vi "Perform Action.vi"(8 "error in":errorcluster, 10 "Input":variant, 11 "Thermometer DAQmx RTD Cont CFG in":refnum<class "Thermometer DAQmx RTD Cont CFG.lvclass">) -> (0 "error out":errorcluster, 2 "Output":variant, 3 "Thermometer DAQmx RTD Cont CFG out":refnum<class "Thermometer DAQmx RTD Cont CFG.lvclass">)   [LabVIEW 2023, in "DAQmx Simulated CFGs.lvlib" / "Thermometer DAQmx RTD Cont CFG.lvclass"]
uses:
  DAQmx/DAQmx Base CFG/DAQmx Base CFG.lvclass/DAQmx Base CFG.ctl
  <vilib>/DAQmx/miscellaneous.llb/DAQmx Fill In Error Info.vi
  Thermometer DAQmx RTD Cont CFG.lvclass
  Thermometer DAQmx RTD Cont CFG.lvclass/Thermometer DAQmx RTD Cont CFG.ctl
  DAQmx/DAQmx Base CFG/DAQmx Base CFG.lvclass
  Thermometer DAQmx RTD Cont CFG/Thermometer DAQmx RTD Cont CFG.lvclass
  <resource>/objmgr/daqmx.rc
  D:/git/HAL/HAL GOOP4/Thermometer/Thermometer DAQmx RTD Cont CFG/Thermometer DAQmx RTD Cont CFG.lvclass
  D:/git/HAL/HAL GOOP4/DAQmx/DAQmx Base CFG/DAQmx Base CFG.lvclass
  D:/git/HAL/HAL GOOP4/CFG Target/CFG Target.lvclass
  D:/git/HAL/HAL GOOP4/Configuration/Configuration Semaphore/CFG Semaphore.lvclass
  D:/git/HAL/HAL GOOP4/Configuration/Configuration JSON/Configuration JSON Base/CFG JSON.lvclass
  D:/git/HAL/HAL GOOP4/Interfaces/IConfigure/IConfigure.lvclass
  D:/git/HAL/HAL GOOP4/Thermometer/Thermometer Simulated CFGs/DAQmx RTD Cont CFG/RTD Cont CFG/Thermometer DAQmx RTD Cont CFG.lvclass
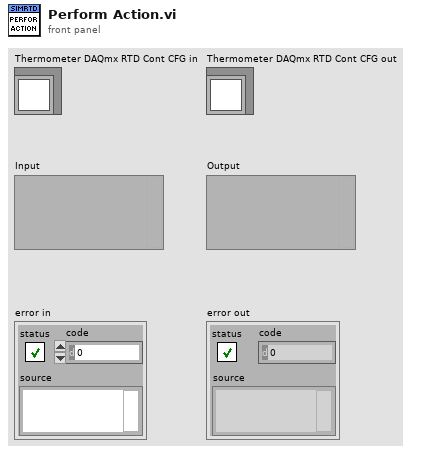
[diagram p1: front panel]
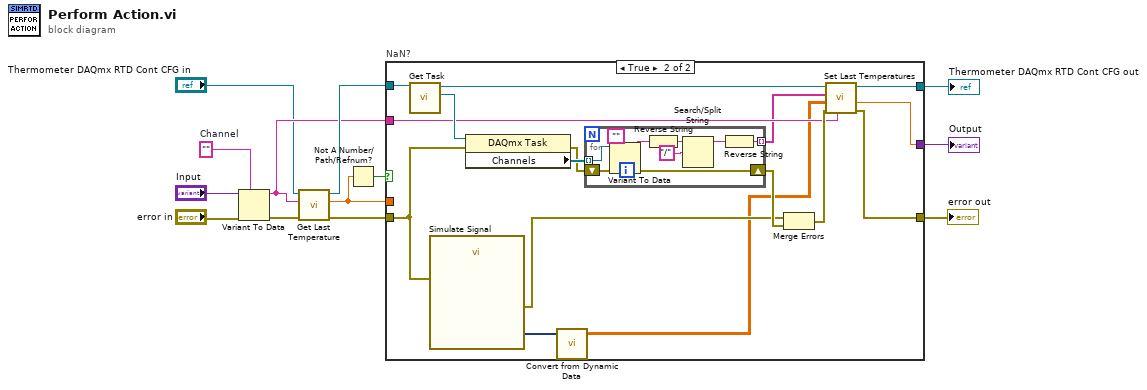
[diagram p0: block diagram]
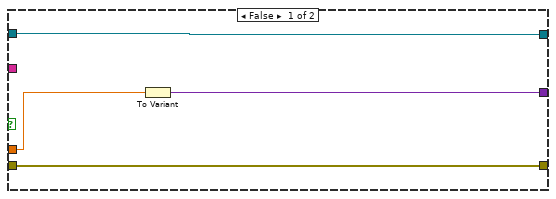
[diagram p2: hidden frame]
diagram:
  w7 = ""  # Channel
  n1 = Variant To Data(error in="error in", type=w7, Variant="Input") -> (data=w8:string, error out=w13:errorcluster)
  n2 = call "Get Last Temperature.vi"("error in"=w13, "Channel"=w8, "Thermometer DAQmx RTD Cont CFG in"="Thermometer DAQmx RTD Cont CFG in") -> ("error out"=w10:errorcluster, "Temperature"=w9:dbl, "Thermometer DAQmx RTD Cont CFG out"=w11:refnum<class "Thermometer DAQmx RTD Cont CFG.lvclass">)  [unwired: 6 in]
  n3 = Not A Number/Path/Refnum?(number/path/refnum=w9) -> (NaN/Path/Refnum?=w12:bool)
  n4 = case "NaN?" shown="True" w12 {
    tunnel: w11 -> [w15 w33]
    tunnel: w10 -> [w14 w21]
    tunnel: [w14 w32] -> w1
    tunnel: [w16 w26] -> w2
    tunnel: [w15 w30] -> w3
    tunnel: w9 -> [w17 _]
    tunnel: w8 -> [_ w27]
    frame False {
      n5 = To Variant(anything=w17) -> (Variant=w16:variant)
    }
    frame True {
      n6 = call "Get Task.vi"("DAQmx Base CFG in"=w33) -> ("Task"=w29:refnum<k21>, "DAQmx Base CFG out"=w31:refnum<class "Thermometer DAQmx RTD Cont CFG.lvclass">)  [unwired: 9 in]
      n7 = call "Simulate Signal"("error in (no error)"=w21) -> ("Sine Temp 50-60"=w19:dynamicdata, "error out"=w20:errorcluster)  [unwired: 13 in]
      n8 = property class="DAQmx Task"(reference=w29, error in=w21) -> (error out=w24:errorcluster, "Channels"=w25:refnum<k21>[])  [unwired: 1 out]
      n9 = call "Convert from Dynamic Data"("Dynamic Data Type"=w19) -> ("Array"=w18:dbl[][])  [unwired: 3 in]
      n10 = for {
        tunnel: w25 -> [w42] mode=indexing
        shift-right: [w37] -> w23
        shift-left: w24 -> [w41]
        tunnel: [w34] -> w22 mode=indexing
        n11 = Variant To Data(error in=w41, type="", Variant=w42) -> (data=w39:string, error out=w37:errorcluster)
        n12 = Reverse String(1:w39) -> (0:w36:string)
        n13 = Search/Split String(string=w36, search string/char (-)="/") -> (substring before match=w35:string)  [unwired: 1 in, 2 out]
        n14 = Reverse String(1:w35) -> (0:w34:string)
      }
      n15 = Merge Errors(w20, w23) -> (w28:errorcluster)
      n16 = call "Set Last Temperatures.vi"("Read Channel Ident"=w27, "error in"=w28, "Temperatures"=w18, "Channel Idents"=w22, "Thermometer DAQmx RTD Cont CFG in"=w31) -> ("error out"=w32:errorcluster, "Temperature"=w26:dbl, "Thermometer DAQmx RTD Cont CFG out"=w30:refnum<class "Thermometer DAQmx RTD Cont CFG.lvclass">)  [unwired: 4 in]
    }
  }
  "error out" <- w1
  "Thermometer DAQmx RTD Cont CFG out" <- w3
  "Output" <- w2
